vi "subscription test.vi"() -> (0 "error out":errorcluster, 1 "remote OK":bool, 2 "local OK":bool, 3 "ALL channels OK":bool)   [LabVIEW 2015, in "tdms logger tests.lvlib"]
uses:
  tdms logger tests.lvlib
  configuration/TDMS datalogger configuration.lvclass/TDMS datalogger configuration.ctl
  <vilib>/NI/Tag Bus/tag/tag descriptor.lvclass/tag descriptor.ctl
  <vilib>/NI/Tag Bus/tag/read tag name.vi
  configuration/Write channels.vi
  configuration/Write channel pattern matches.vi
  configuration/TDMS datalogger configuration.lvclass
  <vilib>/NI/Tag Bus Module Framework/channel/TBM channel.lvclass
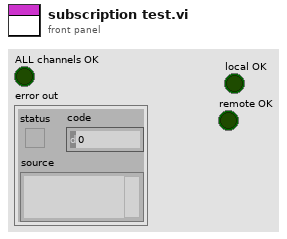
[diagram p1: front panel]
types:
  T1 = cluster{"channel":refnum<class "TBM channel.lvclass">}[]
  T2 = typedef "TBM module configuration.lvclass/channel reservation.ctl" = cluster{"local channel":refnum<class "TBM channel.lvclass">, "remote channel":refnum<class "TBM channel.lvclass">}
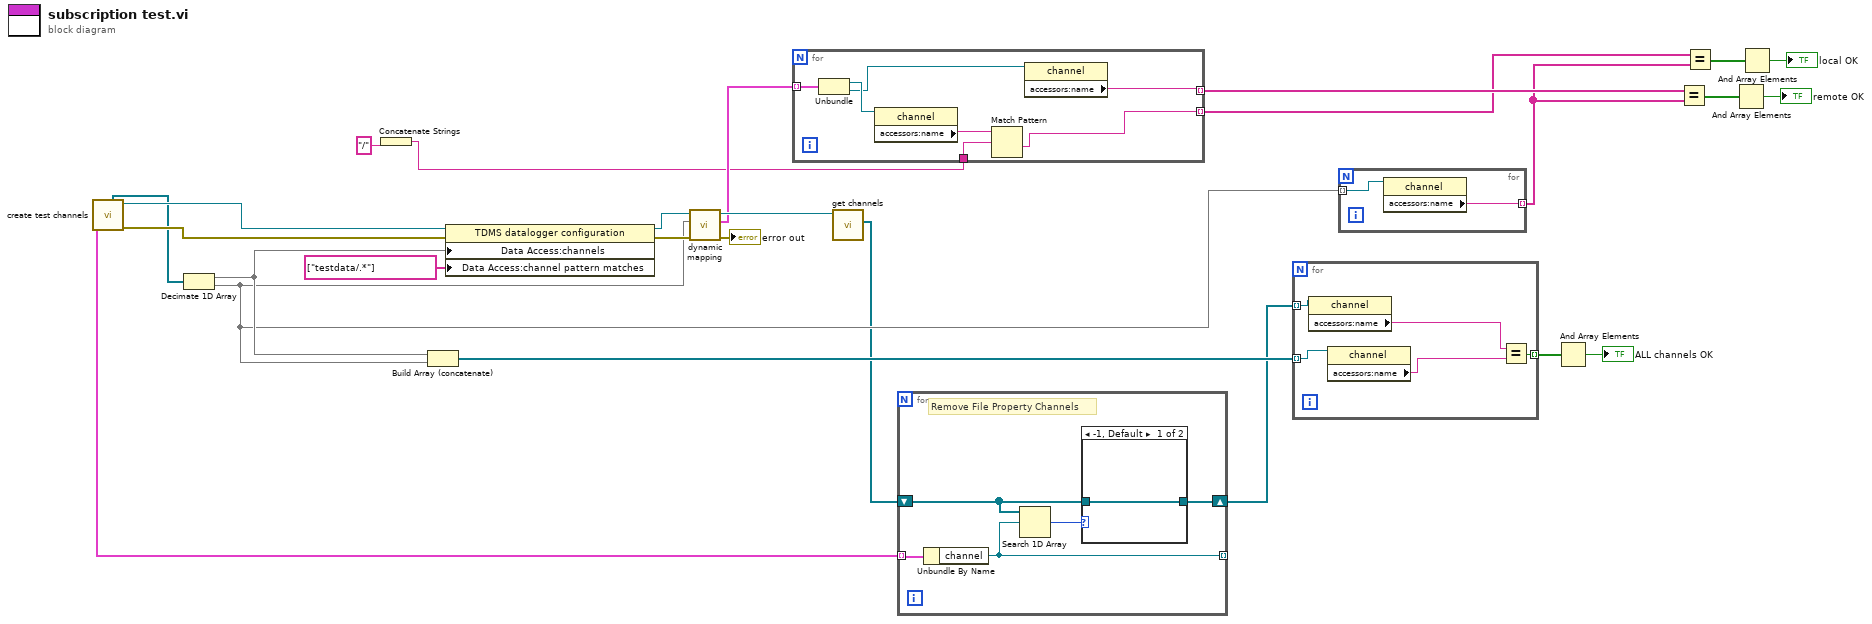
[diagram p0: block diagram]
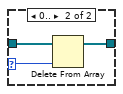
[diagram p2: hidden frame]
diagram:
  n1 = call "create test channels.vi"() -> ("error out"=w6:errorcluster, "TDMS datalogger configuration out"=w7:refnum<class "TDMS datalogger configuration.lvclass">, "chans"=w3:refnum<class "TBM channel.lvclass">[], "Lines"=w4:T1)  [unwired: 3 in, 5 out]
  n2 = Decimate 1D Array(w3) -> (w21:refnum<class "TBM channel.lvclass">[], w5:refnum<class "TBM channel.lvclass">[])
  n3 = Concatenate Strings("/" ("string")) -> (w10:string)
  n4 = Build Array (concatenate)(w21, w5) -> (w20:refnum<class "TBM channel.lvclass">[])
  n5 = property class="TDMS datalogger configuration"(reference=w7, error in=w6, "Data Access:channels"=w21, "Data Access:channel pattern matches"=string[] ["testdata/.*"] ("channel pattern matches")) -> (reference out=w24:refnum<class "TDMS datalogger configuration.lvclass">, error out=w25:errorcluster)
  n6 = call-dynamic "dynamic mapping.vi"("error in"=w25, "channels available"=w5, "module configuration in"=w24) -> ("error out"=→"error out":errorcluster, "reservations"=w17:T2[], "module configuration out"=w22:refnum<class "TDMS datalogger configuration.lvclass">)  [unwired: 6 in]
  n7 = for {
    tunnel: w17 -> [w33] mode=indexing
    tunnel: [w28] -> w14 mode=indexing
    tunnel: [w29] -> w11 mode=indexing
    tunnel: w10 -> [w31]
    n8 = Unbundle(w33) -> ("local channel"=w32:refnum<class "TBM channel.lvclass">, "remote channel"=w27:refnum<class "TBM channel.lvclass">)
    n9 = property class="channel"(reference=w32) -> ("accessors:name"=w30:string)  [unwired: 1 in, 2 out]
    n10 = Match Pattern(string=w30, regular expression=w31) -> (after substring=w29:string)  [unwired: 1 in, 3 out]
    n11 = property class="channel"(reference=w27) -> ("accessors:name"=w28:string)  [unwired: 1 in, 2 out]
  }
  n12 = call-dynamic "get channels.vi"("module configuration in"=w22) -> ("channels"=w2:refnum<class "TBM channel.lvclass">[])  [unwired: 9 in, 1 out]
  n13 = for {
    tunnel: w4 -> [w38] mode=indexing
    tunnel: [w34] -> _ mode=indexing
    shift-right: [w35] -> w1
    shift-left: w2 -> [w36]
    # "Remove File Property Channels"
    n14 = Unbundle By Name(w38) -> ("channel"=w34:refnum<class "TBM channel.lvclass">)
    n15 = Search 1D Array(1D array=w36, element=w34) -> (index of element=w37:i32)  [unwired: 1 in]
    n16 = case shown="-1, Default" w37 {
      selector: w37 -> [_ w42]
      tunnel: w36 -> [w39 w41]
      tunnel: [w39 w40] -> w35
      frame -1, Default {
      }
      frame 0.. {
        n17 = Delete From Array(array=w41, index=w42) -> (array with subset deleted=w40:refnum<class "TBM channel.lvclass">[])  [unwired: 1 in, 1 out]
      }
    }
  }
  n18 = for {
    tunnel: w1 -> [w46] mode=indexing
    tunnel: w20 -> [w45] mode=indexing
    tunnel: [w47] -> w19 mode=indexing
    n19 = property class="channel"(reference=w46) -> ("accessors:name"=w43:string)  [unwired: 1 in, 2 out]
    n20 = property class="channel"(reference=w45) -> ("accessors:name"=w44:string)  [unwired: 1 in, 2 out]
    n21 = Equal?(x=w43, y=w44) -> (x = y?=w47:bool)
  }
  n22 = for {
    tunnel: [w49] -> w8 mode=indexing
    tunnel: w5 -> [w48] mode=indexing
    n23 = property class="channel"(reference=w48) -> ("accessors:name"=w49:string)  [unwired: 1 in, 2 out]
  }
  n24 = And Array Elements(Boolean array=w19) -> (logical AND=→"ALL channels OK":bool)
  n25 = Equal?(x=w14, y=w8) -> (x = y?=w15:bool[])
  n26 = Equal?(x=w11, y=w8) -> (x = y?=w13:bool[])
  n27 = And Array Elements(Boolean array=w15) -> (logical AND=→"remote OK":bool)
  n28 = And Array Elements(Boolean array=w13) -> (logical AND=→"local OK":bool)
